vi "Create Frame Pattern Script.vi"(8 "error in (no error)":errorcluster, 9 "ChipID":u8, 10 "Frame_Data":T1={"Pattern_Name"="", "Operation Mode"=enum."Normal", "BurstLength"=enum."0", "FSN"=0, "Start_Addr"=0, "Data"=[], "R/W?"=enum."Read", "Opcode"=[], "ChipID"=1, "num of wait cycle of read"=0} {"Data" format="%x"; "Start_Addr" format="%x"}, 11 "BML_Frame_ReadData_Compare in":refnum<class "BML_Frame_ReadData_Compare.lvclass">) -> (0 "error out":errorcluster, 3 "BML_Frame_ReadData_Compare out":refnum<class "BML_Frame_ReadData_Compare.lvclass">)   [LabVIEW 2018, in "BML_Frame_ReadData_Compare.lvclass"]
uses:
  BML_Frame_ReadData_Compare.lvclass
  C:/P4 Workspace/PC Client/Solutions/5g_eap/HiSi/trunk/1.0/BML_Pattern_Gen_Refactor/Classes/BML_Frame_Root/BML_Frame_Root.lvclass
  Config_Read/Frame_Data.ctl
  Config_Read/OperationMode.ctl
  Config_Read/BurstLength.ctl
  Config_Read/RW_Option.ctl
  BML_Frame_ReadData_Compare.lvclass/BML_Frame_ReadData_Compare.ctl
  BML_Frame_Root/BML_Frame_Root.lvclass/BML_Frame_Root.ctl
  BML_Frame_Cmd/BML_Frame_Command.lvclass
  BML_Frame_Addr/BML_Frame_Addr.lvclass
  Config_Read/Config_Read_BML.lvclass
  BML_Frame_Root/BML_Frame_Root.lvclass
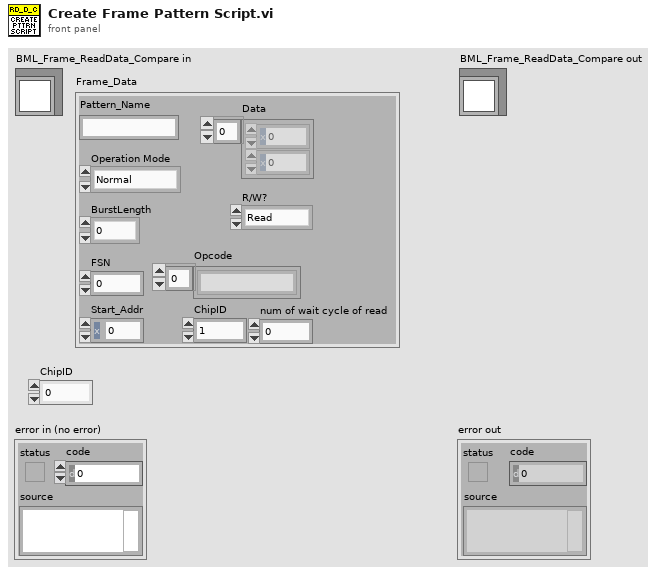
[diagram p1: front panel]
types:
  T1 = typedef "Config_Read_BML.lvclass/Frame_Data.ctl" = cluster{"Pattern_Name":string, "Operation Mode":T2, "BurstLength":T3, "FSN":u8, "Start_Addr":u16, "Data":u8[], "R/W?":T4, "Opcode":string[], "ChipID":u8, "num of wait cycle of read":i8}
  T2 = typedef "Config_Read_BML.lvclass/OperationMode.ctl" = enum8{"Normal", "ImmeEffect", "InitSlaveID", "LoadData"}
  T3 = typedef "Config_Read_BML.lvclass/BurstLength.ctl" = enum8{"0", "2", "3", "4", "5", "8", "16", "32"}
  T4 = typedef "Config_Read_BML.lvclass/RW_Option.ctl" = enum16{"Read", "Write", "R/W"}
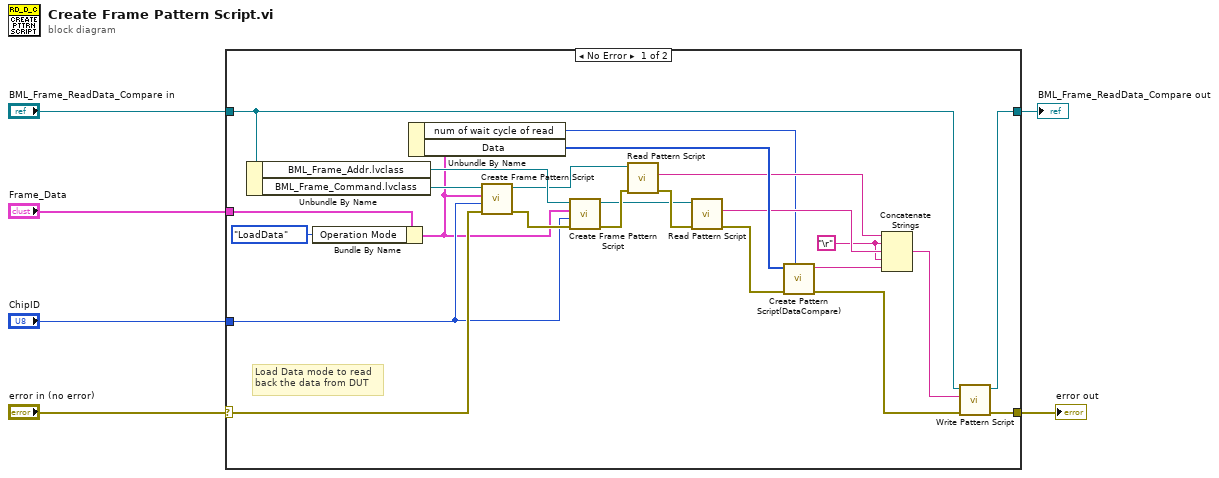
[diagram p0: block diagram]
diagram:
  n1 = case shown="No Error" "error in (no error)" {
    selector: "error in (no error)" -> [w27 w31]
    tunnel: "BML_Frame_ReadData_Compare in" -> [w11 w32]
    tunnel: [w10 w32] -> w4
    tunnel: [w12 w31] -> w3
    tunnel: "Frame_Data" -> [w30 _]
    tunnel: "ChipID" -> [w24 _]
    frame No Error {
      w9 = "\r"
      # "Load Data mode to read\nback the data from DUT"
      n2 = Unbundle By Name(w11) -> ("BML_Frame_Addr.lvclass"=w26:refnum<class "BML_Frame_Addr.lvclass">, "BML_Frame_Command.lvclass"=w28:refnum<class "BML_Frame_Command.lvclass">)
      n3 = Bundle By Name(cluster=w30, "Operation Mode"=OperationMode."LoadData") -> (w19:T1)
      n4 = Unbundle By Name(w19) -> ("num of wait cycle of read"=w7:i8, "Data"=w18:u8[])
      n5 = call-dynamic "Create Frame Pattern Script.vi"("error in (no error)"=w27, "ChipID"=w24, "Frame_Data"=w19, "BML_Frame_Command in"=w28) -> ("error out"=w25:errorcluster, "BML_Frame_Command out"=w23:refnum<class "BML_Frame_Command.lvclass">)  [unwired: 6 in]
      n6 = call-dynamic "Create Frame Pattern Script.vi"("error in (no error)"=w25, "ChipID"=w24, "Frame_Data"=w19, "BML_Frame_Addr in"=w26) -> ("error out"=w22:errorcluster, "BML_Frame_Addr out"=w20:refnum<class "BML_Frame_Addr.lvclass">)  [unwired: 6 in]
      n7 = call "Read Pattern Script.vi"("error in (no error)"=w22, "BML_Frame_Root in"=w23) -> ("error out"=w21:errorcluster, "Pattern Script"=w16:string)  [unwired: 7 in, 1 out]
      n8 = call "Read Pattern Script.vi"("error in (no error)"=w21, "BML_Frame_Root in"=w20) -> ("error out"=w17:errorcluster, "Pattern Script"=w15:string)  [unwired: 7 in, 1 out]
      n9 = call "Create Pattern Script(DataCompare).vi"("Num of wait cycle for read"=w7, "error in (no error)"=w17, "Data"=w18) -> ("error out"=w13:errorcluster, "String"=w8:string)  [unwired: 7 in]
      n10 = Concatenate Strings(w16, w9, w15, w9, w8) -> (w14:string)
      n11 = call "Write Pattern Script.vi"("error in (no error)"=w13, "Pattern Script"=w14, "BML_Frame_Root in"=w11) -> ("error out"=w12:errorcluster, "BML_Frame_Root out"=w10:refnum<class "BML_Frame_ReadData_Compare.lvclass">)  [unwired: 7 in]
    }
    frame Error {
    }
  }
  "error out" <- w3
  "BML_Frame_ReadData_Compare out" <- w4
